vi "Interface Default Data.vi"() -> (2 "Interface Default Data":variant=variant(cluster{} {}))   [LabVIEW 2017, in "Composition.lvlib"]
doc: "Returns the default data of an interface class."
uses:
  Composition.lvlib
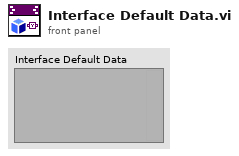
[diagram p1: front panel]
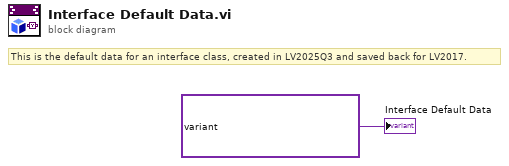
[diagram p0: block diagram]
diagram:
  # "This is the default data for an interface class, created in LV2025Q3 and saved back for LV2017."
  "Interface Default Data" <- variant(cluster{} {}) ("Class Default Data")
